vi "Rotation Matrix to Euler Angles.vi"(1 "rotation matrix":T2) -> (0 "euler angles":T1)   [LabVIEW 2017, in "NI_Kinematics.lvlib"]
doc: "Converts the <B>rotation matrix</B> you specify to Z, X, and Z Euler angles.\n\n<B>.m file:</B> tr2eul"
uses:
  <vilib>/robotics/Kinematics/NI_Kinematics.lvlib
  <vilib>/Analysis/Matrix/Datatypes/RealMatrix.ctl
  <vilib>/Analysis/NI_AALPro.lvlib
  <vilib>/Analysis/Matrix/NI_Matrix.lvlib
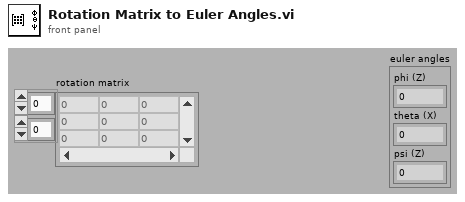
[diagram p1: front panel]
types:
  T1 = cluster{"phi (Z)":dbl, "theta (X)":dbl, "psi (Z)":dbl}
  T2 = typedef "NI_Matrix.lvlib/RealMatrix.ctl" = dbl[][]
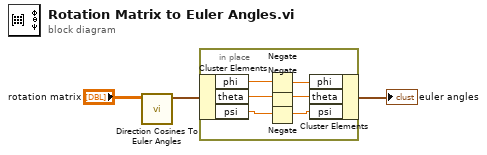
[diagram p0: block diagram]
diagram:
  n1 = call <vilib>:"Direction Cosines To Euler Angles.vi"("Direction Cosines"="rotation matrix") -> ("Euler Angles"=w2:cluster{"phi":dbl, "theta":dbl, "psi":dbl})  [unwired: 9 in, 1 out]
  n2 = in-place {
    n3 = in-place-cluster #1(w2) -> ("phi"=w9:dbl, "theta"=w7:dbl, "psi"=w5:dbl)
    n4 = Negate(x=w9) -> (-x=w8:dbl)
    n5 = Negate(x=w7) -> (-x=w6:dbl)
    n6 = Negate(x=w5) -> (-x=w4:dbl)
    n7 = in-place-cluster #1("phi"=w8, "theta"=w6, "psi"=w4) -> (→"euler angles":cluster{"phi":dbl, "theta":dbl, "psi":dbl})
  }
